vi "format Logstring.vi"(11 "LogRecord in":refnum<class "LogRecord.lvclass">) -> (3 "LogLine":string)   [LabVIEW 2023, in "horiba.lvlib" / "LiveLogger.lvlib"]
uses:
  LiveLogger.lvlib
  <vilib>/Hampel Software Engineering/HSE Logger/LogRecord/LogRecord.lvclass
  <vilib>/Hampel Software Engineering/HSE Logger/LogRecord/LogRecord.lvclass/LogRecord.ctl
  <vilib>/Hampel Software Engineering/HSE Logger/LogRecord/Get Level.vi
  <vilib>/Hampel Software Engineering/HSE Logger/Formatter/HSE_v2_Formatter/HSE_v2_Formatter.lvclass
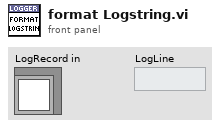
[diagram p1: front panel]
types:
  T1 = typedef "hse-logger.lvlib/LogLevel.ctl" = enum16{"DEBUG", "INFO", "WARNING", "ERROR", "CRITICAL"}
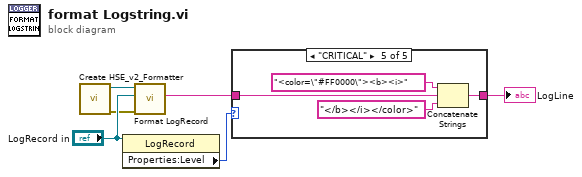
[diagram p0: block diagram]
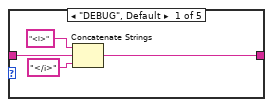
[diagram p2: hidden frame]
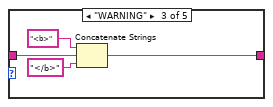
[diagram p4: hidden frame]
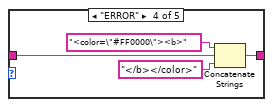
[diagram p5: hidden frame]
diagram:
  n1 = call <vilib>:"Create HSE_v2_Formatter.vi"() -> ("error out"=w2:errorcluster, "HSE_v2_Formatter out"=w6:refnum<class "HSE_v2_Formatter.lvclass">)  [unwired: 10 in]
  n2 = property class="LogRecord"(reference="LogRecord in") -> ("Properties:Level"=w3:T1)  [unwired: 1 in, 2 out]
  n3 = call-dynamic "Format LogRecord.vi"("error in"=w2, "LogRecord"="LogRecord in", "HSE_v2_Formatter in"=w6) -> ("LogLine"=w4:string)  [unwired: 7 in, 1 out]
  n4 = case shown="\"CRITICAL\"" w3 {
    tunnel: w4 -> [w8 w11 w13 w17 w21]
    tunnel: [w7 w11 w12 w16 w20] -> w1
    frame "DEBUG", Default {
      n5 = Concatenate Strings("<i>" ("string"), w8, "</i>" ("string")) -> (w7:string)
    }
    frame "INFO" {
    }
    frame "WARNING" {
      n6 = Concatenate Strings("<b>" ("string"), w13, "</b>" ("string")) -> (w12:string)
    }
    frame "ERROR" {
      n7 = Concatenate Strings("<color=\"#FF0000\"><b>" ("string"), w17, "</b></color>" ("string")) -> (w16:string)
    }
    frame "CRITICAL" {
      n8 = Concatenate Strings("<color=\"#FF0000\"><b><i>" ("string"), w21, "</b></i></color>" ("string")) -> (w20:string)
    }
  }
  "LogLine" <- w1
